vi "standard_cmd_read.vi"(5 "COM":bool, 6 "error in (no error)":errorcluster, 7 "VISA name":refnum<visa-resource-name>, 8 "data":u8[](array[numeric]), 9 "dwLen":u32 format="%.0x", 10 "dwAddr":u32 format="%.0x", 11 "cmd_std_header_t":T1) -> (2 "return":i32, 3 "data out":u8[](array[numeric]), 4 "error out":errorcluster)   [LabVIEW 2016]
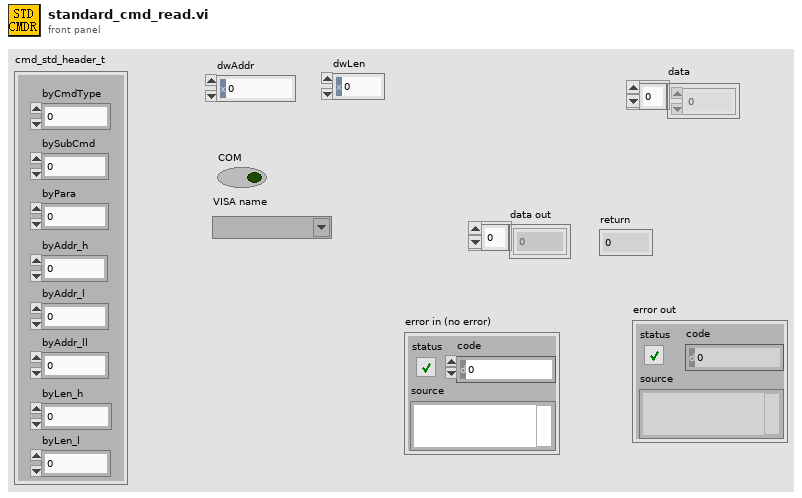
[diagram p1: front panel]
types:
  T1 = cluster{"byCmdType":u8, "bySubCmd":u8, "byPara":u8, "byAddr_h":u8, "byAddr_l":u8, "byAddr_ll":u8, "byLen_h":u8, "byLen_l":u8}
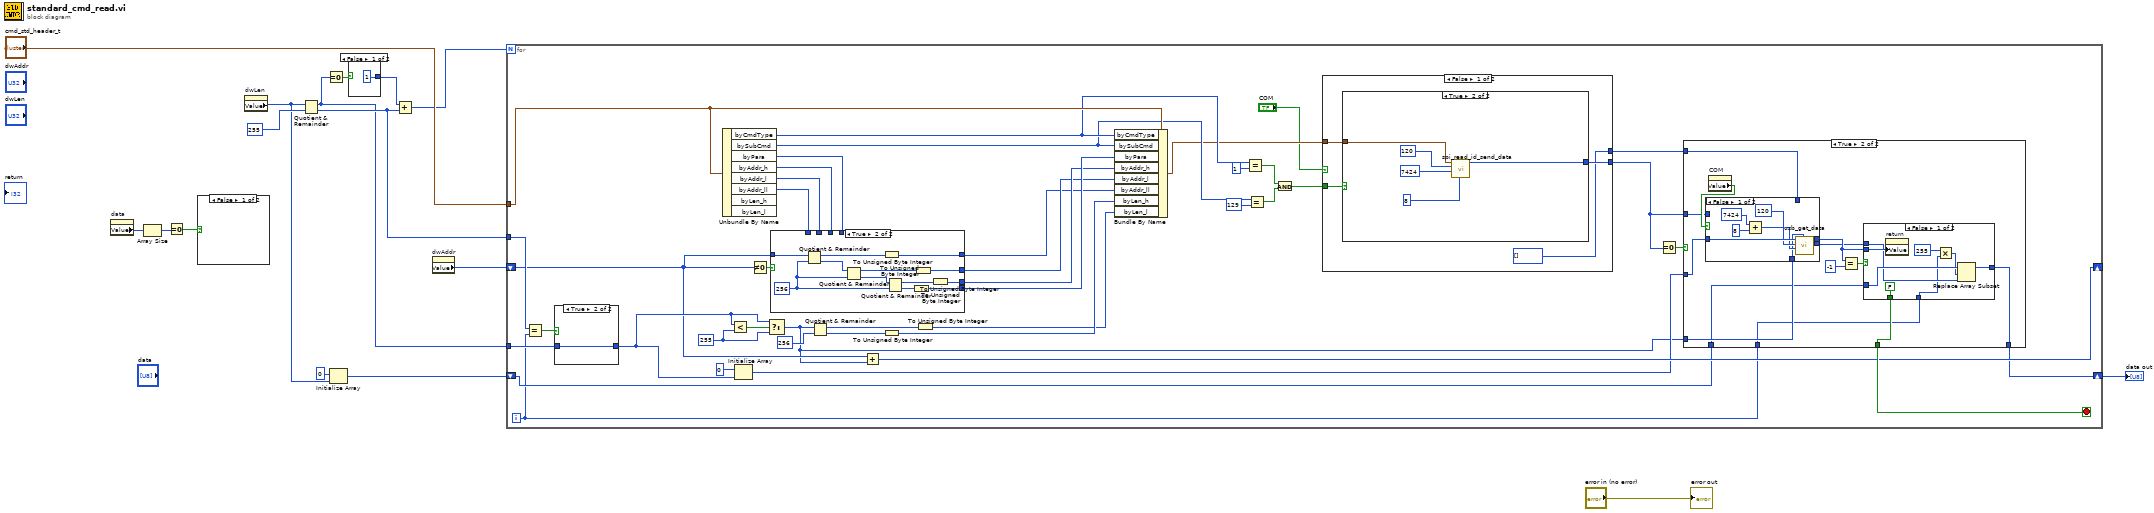
[diagram p0: block diagram]
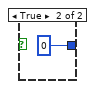
[diagram p2: hidden frame]
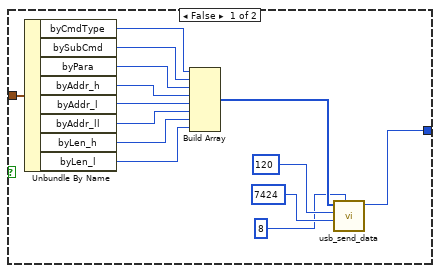
[diagram p3: hidden frame]
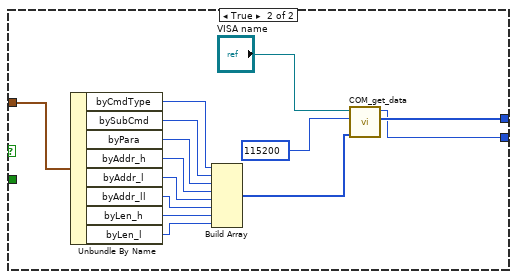
[diagram p4: hidden frame]
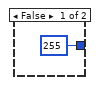
[diagram p5: hidden frame]
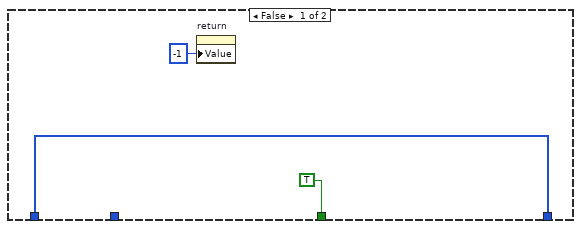
[diagram p6: hidden frame]
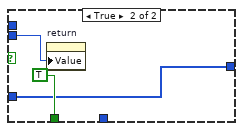
[diagram p8: hidden frame]
diagram:
  n1 = property on="data" class="Arr (strict)"() -> ("Value"=w16:u8[])  [unwired: 2 in, 2 out]
  n2 = Array Size(array=w16) -> (size(s)=w14:i32)
  n3 = Equal To 0?(x=w14) -> (x = 0?=w15:bool)
  n4 = case shown="False" w15 {
    frame False {
    }
    frame True {
    }
  }
  n5 = property on="dwLen" class="DigNum (strict)"() -> ("Value"=w4:u32)  [unwired: 2 in, 2 out]
  n6 = Quotient & Remainder(x=w4, y=u32 255) -> (x-y*floor(x/y)=w7:u32, floor(x/y)=w8:u32)
  n7 = Equal To 0?(x=w7) -> (x = 0?=w11:bool)
  n8 = Initialize Array(u8 0, w4) -> (w2:u8[])
  n9 = case shown="False" w11 {
    tunnel: [u32 1 u32 0] -> w10
    frame False {
    }
    frame True {
    }
  }
  n10 = Add(x=w10, y=w8) -> (x+y=w9:u32)
  n11 = property on="dwAddr" class="DigNum (strict)"() -> ("Value"=w6:u32)  [unwired: 2 in, 2 out]
  n12 = for {
    N: w9 -> [_]
    tunnel: "cmd_std_header_t" -> [w57]
    tunnel: w8 -> [w32]
    tunnel: w7 -> [w31]
    shift-right: [w23] -> w5
    shift-left: w2 -> [w24]
    shift-right: [w27] -> _
    shift-left: w6 -> [w28]
    i -> [w22]
    stop <- w34 stop-if-true
    w59 = u32 255 ("f")
    n13 = Equal?(x=w32, y=w22) -> (x = y?=w33:bool)
    n14 = case shown="True" w33 {
      tunnel: w31 -> [_ w99]
      tunnel: [u32 255 w99] -> w29
      frame False {
      }
      frame True {
      }
    }
    n15 = Unbundle By Name(w57) -> ("byCmdType"=w43:u8, "bySubCmd"=w41:u8, "byPara"=w47:u8, "byAddr_h"=w46:u8, "byAddr_l"=w45:u8, "byAddr_ll"=w44:u8)  [unwired: 2 out]
    n16 = Less?(x=w29, y=w59) -> (x < y?=w60:bool)
    n17 = Initialize Array(u8 0 ("element"), w29) -> (w26:u8[])
    n18 = Not Equal To 0?(x=w28) -> (x != 0?=w48:bool)
    n19 = Select(t=w29, s=w60, f=w59) -> (s? t:f=w25:u32)
    n20 = case shown="True" w48 {
      tunnel: w28 -> [_ w152]
      tunnel: [w140 w147] -> w56
      tunnel: [w139 w143] -> w51
      tunnel: [w138 w142] -> w50
      tunnel: [w137 w141] -> w49
      tunnel: w47 -> [w140 _]
      tunnel: w46 -> [w139 _]
      tunnel: w45 -> [w138 _]
      tunnel: w44 -> [w137 _]
      frame False {
      }
      frame True {
        w149 = u32 256 ("y")
        n21 = Quotient & Remainder(x=w152, y=w149) -> (x-y*floor(x/y)=w144:u32, floor(x/y)=w151:u32)
        n22 = Quotient & Remainder(x=w151, y=w149) -> (x-y*floor(x/y)=w145:u32, floor(x/y)=w150:u32)
        n23 = To Unsigned Byte Integer(number=w144) -> (unsigned 8bit integer=w141:u8)
        n24 = Quotient & Remainder(x=w150, y=w149) -> (x-y*floor(x/y)=w146:u32, floor(x/y)=w148:u32)
        n25 = To Unsigned Byte Integer(number=w148) -> (unsigned 8bit integer=w147:u8)
        n26 = To Unsigned Byte Integer(number=w145) -> (unsigned 8bit integer=w142:u8)
        n27 = To Unsigned Byte Integer(number=w146) -> (unsigned 8bit integer=w143:u8)
      }
    }
    n28 = Quotient & Remainder(x=w25, y=u32 256) -> (x-y*floor(x/y)=w54:u32, floor(x/y)=w55:u32)
    n29 = Add(x=w28, y=w25) -> (x+y=w27:u32)
    n30 = To Unsigned Byte Integer(number=w55) -> (unsigned 8bit integer=w53:u8)
    n31 = To Unsigned Byte Integer(number=w54) -> (unsigned 8bit integer=w52:u8)
    n32 = Bundle By Name(cluster=w57, "byCmdType"=w43, "bySubCmd"=w41, "byPara"=w56, "byAddr_h"=w51, "byAddr_l"=w50, "byAddr_ll"=w49, "byLen_h"=w53, "byLen_l"=w52) -> (w36:T1)
    n33 = Equal?(x=w43, y=u8 1) -> (x = y?=w39:bool)
    n34 = Equal?(x=w41, y=u8 129) -> (x = y?=w38:bool)
    n35 = And(x=w39, y=w38) -> (x .and. y?=w37:bool)
    n36 = case shown="False" "COM" {
      tunnel: w37 -> [w64 _]
      tunnel: w36 -> [w63 w95]
      tunnel: [w62 w84] -> w19
      tunnel: [u8[] [] ("data out") w85] -> w20
      frame False {
        n37 = case shown="True" w64 {
          tunnel: w63 -> [w75 w83]
          tunnel: [w76 w80] -> w62
          frame False {
            n38 = Unbundle By Name(w75) -> ("byCmdType"=w74:u8, "bySubCmd"=w73:u8, "byPara"=w72:u8, "byAddr_h"=w71:u8, "byAddr_l"=w70:u8, "byAddr_ll"=w69:u8, "byLen_h"=w68:u8, "byLen_l"=w67:u8)
            n39 = Build Array(w74, w73, w72, w71, w70, w69, w68, w67) -> (w66:u8[])
            n40 = call "usb_send_data.vi"("byVdCmdHeaderLen"=u16 8, "I2C_VD_BUFFER_RW"=u16 7424, "I2C_SLAVE_ID"=u8 120, "data"=w66) -> ("return"=w76:i32)  [unwired: 6 in, 1 out]
          }
          frame True {
            n41 = call "spi_read_id_send_data.vi"("byVdCmdHeaderLen"=u16 8, "I2C_VD_BUFFER_RW"=u16 7424, "I2C_SLAVE_ID"=u8 120, "cmd_std_header_t"=w83) -> ("return"=w80:i32)  [unwired: 6 in, 1 out]
          }
        }
      }
      frame True {
        n42 = Unbundle By Name(w95) -> ("byCmdType"=w94:u8, "bySubCmd"=w93:u8, "byPara"=w92:u8, "byAddr_h"=w91:u8, "byAddr_l"=w90:u8, "byAddr_ll"=w89:u8, "byLen_h"=w88:u8, "byLen_l"=w87:u8)
        n43 = Build Array(w94, w93, w92, w91, w90, w89, w88, w87) -> (w86:u8[])
        n44 = call "COM_get_data.vi"("data"=w86, "baud rate (9600)"=u32 115200, "VISA name"="VISA name") -> ("data out"=w85:u8[], "return"=w84:i32)  [unwired: 7 in]
      }
    }
    n45 = Equal To 0?(x=w19) -> (x = 0?=w35:bool)
    n46 = case shown="True" w35 {
      tunnel: [TRUE w111] -> w34
      tunnel: w26 -> [_ w115]
      tunnel: w25 -> [_ w114]
      tunnel: w24 -> [w100 w109]
      tunnel: [w100 w106] -> w23
      tunnel: w22 -> [_ w107]
      tunnel: w20 -> [_ w104]
      tunnel: w19 -> [_ w103]
      frame False {
        n47 = property on="return" class="DigNum (strict)"("Value"=-1 ("return")) -> ()  [unwired: 2 in, 2 out]
      }
      frame True {
        n48 = property on="COM" class="Bool (strict)"() -> ("Value"=w105:bool)  [unwired: 2 in, 2 out]
        n49 = case shown="False" w105 {
          tunnel: w115 -> [w123 _]
          tunnel: w114 -> [w116 _]
          tunnel: [w118 w124] -> w110
          tunnel: [w117 w125] -> w108
          tunnel: w104 -> [_ w125]
          tunnel: w103 -> [_ w124]
          frame False {
            n50 = Add(x=u16 7424 ("I2C_VD_BUFFER_RW"), y=u16 8) -> (x+y=w119:u16)
            n51 = call "usb_get_data.vi"("byVdCmdHeaderLen"=w116, "I2C_VD_BUFFER_RW"=w119, "I2C_SLAVE_ID"=u8 120, "data"=w123) -> ("data out"=w117:u8[], "return"=w118:i32)  [unwired: 5 in, 1 out]
          }
          frame True {
          }
        }
        n52 = Equal?(x=w110, y=-1) -> (x = y?=w113:bool)
        n53 = case shown="False" w113 {
          tunnel: [FALSE TRUE] -> w111
          tunnel: w110 -> [w132 w135]
          tunnel: w109 -> [w131 w134]
          tunnel: w108 -> [w130 _]
          tunnel: w107 -> [w128 _]
          tunnel: [w126 w134] -> w106
          frame False {
            n54 = property on="return" class="DigNum (strict)"("Value"=w132) -> ()  [unwired: 2 in, 2 out]
            n55 = Multiply(x=255, y=w128) -> (x*y=w127:i32)
            n56 = Replace Array Subset(array=w131, new element=w130, index=w127) -> (w126:u8[])
          }
          frame True {
            n57 = property on="return" class="DigNum (strict)"("Value"=w135) -> ()  [unwired: 2 in, 2 out]
          }
        }
      }
    }
  }
  "data out" <- w5
  "error out" <- "error in (no error)"
